vi "Set Splitter Size (Core).vi"(8 "error in (no error)":errorcluster, 10 "Size":i32, 11 "Splitter in":refnum<class "Splitter.lvclass">) -> (0 "error out":errorcluster, 3 "Splitter out":refnum<class "Splitter.lvclass">)   [LabVIEW 2019, in "Splitter.lvclass"]
uses:
  <resource>/dialog/QuickDrop/plugins/PaneRelief/Classes/Splitter/Splitter.lvclass
  <resource>/dialog/QuickDrop/plugins/PaneRelief/Classes/Splitter/Splitter.lvclass/Splitter.ctl
  8fc9ccee-7f60-4d20-af5d-90eb1da01e0b.vi
  8e0fcfb2-f584-410e-8456-2735d8fed526.vi
  <resource>/dialog/QuickDrop/plugins/PaneRelief/Low-Level VI Manipulation/Find Resource by Type (String).vi
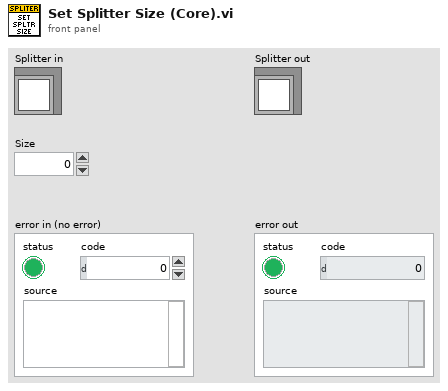
[diagram p1: front panel]
types:
  T1 = typedef "Resource Array.ctl" = T2[]
  T2 = typedef "Resource.ctl" = cluster{"type":u32, "id":i32, "name":string, "binary data":string}
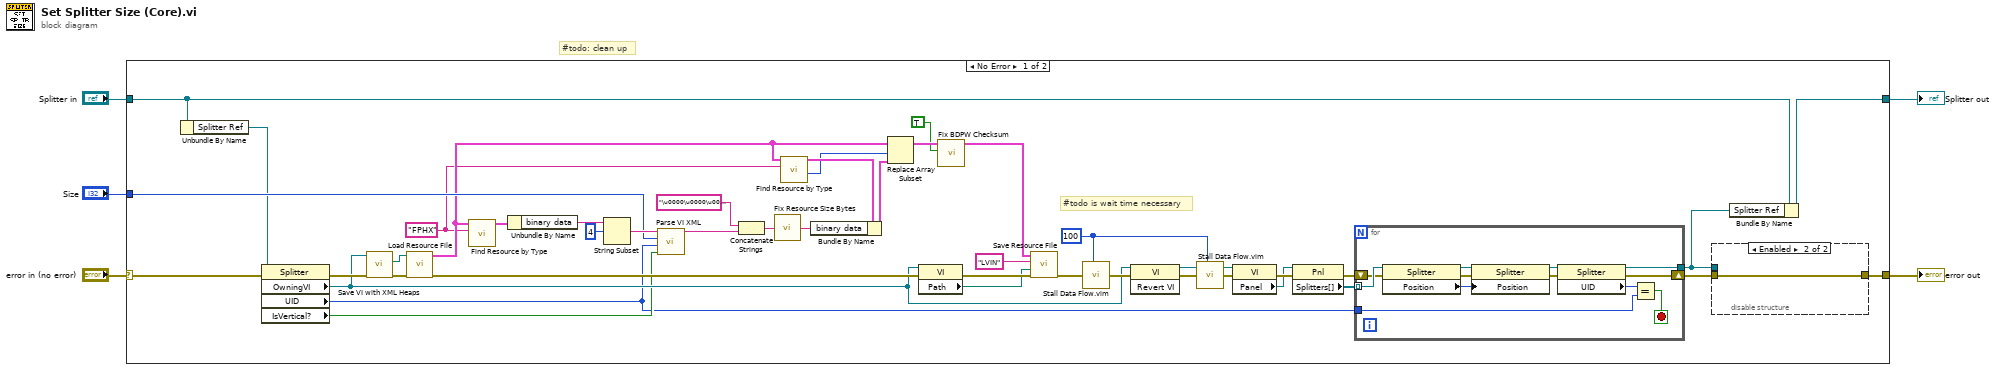
[diagram p0: block diagram]
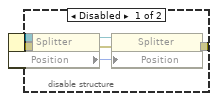
[diagram p2: hidden frame]
diagram:
  # "#todo: clean up"
  n1 = case shown="No Error" "error in (no error)" {
    selector: "error in (no error)" -> [w44 w69]
    tunnel: [w19 w69] -> w4
    tunnel: [w8 w70] -> w2
    tunnel: "Splitter in" -> [w7 w70]
    tunnel: "Size" -> [w41 _]
    frame No Error {
      w24 = u32 100 ("milliseconds to wait")
      w20 = "FPHX"
      # "#todo is wait time necessary"
      n2 = Unbundle By Name(w7) -> ("Splitter Ref"=w9:refnum<vi>)
      n3 = property class="Splitter"(reference=w9, error in=w44) -> (error out=w42:errorcluster, "OwningVI"=w22:refnum<vi>, "UID"=w11:i32, "IsVertical?"=w12:bool)  [unwired: 1 out]
      n4 = call <resource>:"Save VI with XML Heaps.vi"("error in (no error)"=w42, "VI Refnum In"=w22) -> ("error out"=w45:errorcluster, "VI Path out"=w49:path)  [unwired: 7 in, 1 out]
      n5 = call <resource>:"Load Resource File.vi"("error in (no error)"=w45, "Resource file"=w49) -> ("error out"=w31:errorcluster, "Resources"=w29:T1)  [unwired: 7 in, 1 out]
      n6 = call-poly <resource>:"Find Resource by Type.vi"("Resource Type"=w20, "Resources"=w29) -> ("Resource"=w46:T2)  [unwired: 7 in, 2 out]
      n7 = Unbundle By Name(w46) -> ("binary data"=w47:string)
      n8 = String Subset(string=w47, offset (0)=4) -> (substring=w43:string)  [unwired: 1 in]
      n9 = call <resource>:"Parse VI XML.vi"("Is Vertical?"=w12, "UID"=w11, "New Size"=w41, "VI XML"=w43) -> ("VI XML With New Size"=w30:string)  [unwired: 6 in, 1 out]
      n10 = Concatenate Strings("\u0000\u0000\u0000\u0000", w30) -> (w39:string)
      n11 = call <resource>:"Fix Resource Size Bytes.vi"("Data In"=w39) -> ("Data Out"=w38:string)
      n12 = call-poly <resource>:"Find Resource by Type.vi"("Resource Type"=w20, "Resources"=w29) -> ("Index"=w36:i32, "Resource"=w37:T2)  [unwired: 7 in, 1 out]
      n13 = Bundle By Name(cluster=w37, "binary data"=w38) -> (w35:T2)
      n14 = Replace Array Subset(array=w29, new element=w35, index=w36) -> (w34:T1)
      n15 = property class="VI"(reference=w22, error in=w31) -> (error out=w27:errorcluster, "Path"=w26:path)  [unwired: 1 out]
      n16 = call <resource>:"Fix BDPW Checksum.vi"("Only fix 3rd hash (F)"=TRUE, "Resources in"=w34) -> ("Resources out"=w33:T1)  [unwired: 9 in]
      n17 = call <resource>:"Save Resource File.vi"("error in (no error)"=w27, "Path"=w26, "File type"="LVIN", "Resources"=w33) -> ("error out"=w25:errorcluster)  [unwired: 7 in]
      n18 = call "Stall Data Flow.vim"("value in"=w25, "milliseconds to wait"=w24) -> ("value out"=w23:errorcluster)  [unwired: 1 out]
      n19 = invoke class="VI" method="Revert VI"(reference=w22, error in=w23) -> (reference out=w18:refnum<vi>, error out=w21:errorcluster)  [unwired: 1 in, 1 out]
      n20 = call "Stall Data Flow.vim"("value in"=w21, "milliseconds to wait"=w24) -> ("value out"=w15:errorcluster)  [unwired: 1 out]
      n21 = property class="VI"(reference=w18, error in=w15) -> (error out=w17:errorcluster, "Panel"=w16:refnum<vi>)  [unwired: 1 out]
      n22 = property class="Pnl"(reference=w16, error in=w17) -> (error out=w14:errorcluster, "Splitters[]"=w13:refnum<vi>[])  [unwired: 1 out]
      n23 = for {
        tunnel: w13 -> [w59] mode=indexing
        tunnel: w11 -> [w67]
        shift-right: [w65] -> w10
        shift-left: w14 -> [w57]
        tunnel: [w64] -> w6
        stop <- w66 stop-if-true
        n24 = property class="Splitter"(reference=w59, error in=w57) -> (reference out=w62:refnum<vi>, error out=w63:errorcluster, "Position"=w61:i32)
        n25 = property class="Splitter"(reference=w62, error in=w63, "Position"=w61) -> (reference out=w60:refnum<vi>, error out=w58:errorcluster)
        n26 = property class="Splitter"(reference=w60, error in=w58) -> (reference out=w64:refnum<vi>, error out=w65:errorcluster, "UID"=w68:i32)
        n27 = Equal?(x=w68, y=w67) -> (x = y?=w66:bool)
      }
      n28 = disable-structure shown="Enabled" {
        disable-tunnel: [w52 w56] -> w19
        disable-tunnel: w10 -> [w51 w56]
        disable-tunnel: w6 -> [w50 _]
        frame Disabled {
          n29 = property class="Splitter"(reference=w50, error in=w51) -> (reference out=w54:refnum<vi>, error out=w53:errorcluster, "Position"=w55:i32)
          n30 = property class="Splitter"(reference=w54, error in=w53, "Position"=w55) -> (error out=w52:errorcluster)  [unwired: 1 out]
        }
        frame Enabled {
        }
      }
      n31 = Bundle By Name(cluster=w7, "Splitter Ref"=w6) -> (w8:refnum<class "Splitter.lvclass">)
    }
    frame Error {
    }
  }
  "error out" <- w4
  "Splitter out" <- w2
